vi "RenameReadEvents.vi"(1 "DAQ.Read":refnum<user-event>[](array[refnum])) -> (0 "DAQ.Read":refnum<user-event>[](array[refnum]))   [LabVIEW 2016, in "DAQ_Manager.lvclass"]
uses:
  DAQ_Manager.lvclass
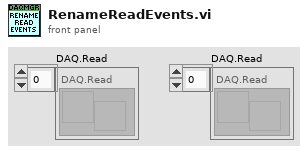
[diagram p1: front panel]
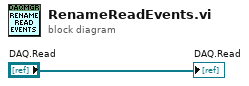
[diagram p0: block diagram]
diagram:
  "DAQ.Read" <- "DAQ.Read"
